vi "Agilent 3458 Acquire Single(Math) Measurement.vi"() -> ()   [LabVIEW 2020, in "3458A Basic Driver.lvlib"]
doc: "Shows how to configure and take a single measurement with the math scale function applied to that measurement."
uses:
  3458A Basic Driver.lvlib
  Public/Data/Read Measurement(Single Point).vi
panel:
  in  "Manual Range (1.00)":dbl=1.0 format="%_3g"
  out "Measurement":dbl
  in  "Scale Value (1.00)":dbl=1.0 format="%_3g"
  in  "Auto Range (1:ON)":u16(ring)=1 items=["OFF", "ON", "ONCE"]
  in  "Trigger Type (0:Auto)":u16(ring) items=["Auto", "External", "Level", "Line", "Synchronous"]
  in  "Manual Resolution (2: 6.5 digits)":enum16{"4.5", "5.5", "6.5", "7.5", "8.5"}(ring)=enum."6.5"
  in  "VISA resource name":refnum<visa-resource-name>
  in  "Frequency Source (3: ACV)":u16(ring)=3 items=["ACDCI", "ACDCV", "ACI", "ACV"]
  in  "Function (0: DC Voltage)":u16(ring) items=["DC Voltage", "AC Voltage", "AC + DC Voltage", "DC Current", "AC Current", "AC + DC Current", "2-Wire Resistance", "4-Wire Resistance", "Frequency", "Period", "Direct Sampling DC", "Direct Sampling AC"]
  # "(c) 2007  National Instruments.  ALL RIGHTS RESERVED."
  # "Scale Function"
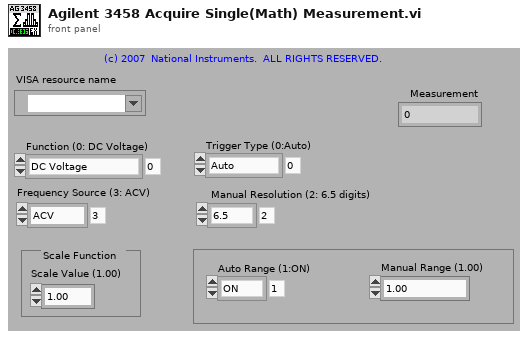
[diagram p1: front panel]
types:
  T1 = enum16{"CRTD85", "CRTD92", "CTHRM", "CTHRM2K", "CTHRM10K", "dB", "dBm", "Filter", "FRTD85", "FRTD92", "FTHRM", "FTHRM2K", "FTHRM10K", "None", "Null", "Pass/Fail", "Percent", "RMS", "Scale", "Statistics"}
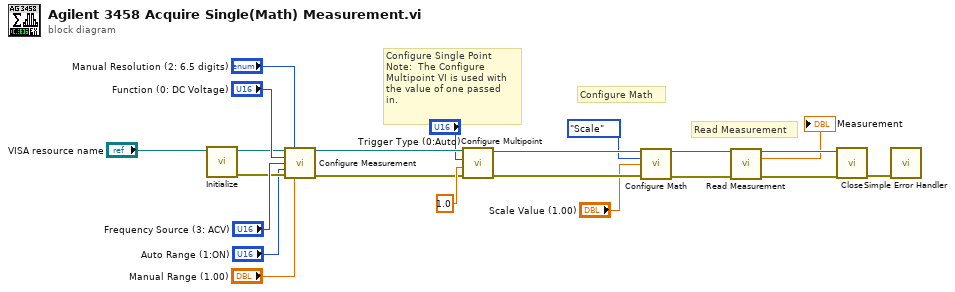
[diagram p0: block diagram]
diagram:
  # "Configure Single Point\nNote:  The Configure \nMultipoint VI is used with\nthe value of one passed\nin."
  # "Read Measurement"
  # "Configure Math"
  n1 = call "Initialize.vi"("VISA resource name"="VISA resource name") -> ("error out"=w10:errorcluster, "VISA resource name out"=w11:refnum<visa-resource-name>)  [unwired: 8 in, 1 out]
  n2 = call "Configure Measurement.vi"("VISA resource name"=w11, "Manual Resolution (2: 6.5 digits)"="Manual Resolution (2: 6.5 digits)", "Function (0: DC Voltage)"="Function (0: DC Voltage)", "Frequency Source (3: AC Voltage)"="Frequency Source (3: ACV)", "Auto Range (1:ON)"="Auto Range (1:ON)", "error in (no error)"=w10, "Manual Range (1.00)"="Manual Range (1.00)") -> ("VISA resource name out"=w15:refnum<visa-resource-name>, "error out"=w14:errorcluster)  [unwired: 7 in]
  n3 = call "Configure Multipoint.vi"("error in (no error)"=w14, "Sample Count (1)"=1.0, "Trigger Type (0:Auto)"="Trigger Type (0:Auto)", "VISA resource name"=w15) -> ("error out"=w12:errorcluster, "VISA resource name out"=w13:refnum<visa-resource-name>)  [unwired: 6 in]
  n4 = call "Configure Math.vi"("VISA resource name"=w13, "Operation (13:None)"=T1."Scale", "Scale Value (1.00)"="Scale Value (1.00)", "error in (no error)"=w12) -> ("VISA resource name out"=w22:refnum<visa-resource-name>, "error out"=w21:errorcluster)  [unwired: 10 in]
  n5 = call-poly "Read Measurement.vi"("VISA resource name"=w22, "error in (no error)"=w21) -> ("VISA resource name out"=w9:refnum<visa-resource-name>, "Measurement"=→"Measurement":dbl, "error out"=w8:errorcluster)  [unwired: 11 in]
  n6 = call "Close.vi"("error in (no error)"=w8, "VISA resource name"=w9) -> ("error out"=w20:errorcluster)  [unwired: 9 in]
  n7 = call <vilib>:"Simple Error Handler.vi"("error in (no error)"=w20) -> ()  [unwired: 4 in, 5 out]
